vi "copy_from_wrapper.vi"() -> ()   [LabVIEW 2019]
panel:
  in  "Interrupt Run":bool
  out "CMD Error":string
  out "CMD Output":string
  in  "CMD Output":bool
  in  "Help Button":bool
  out "Output Files Path":path caption="selected path"
  in  "Open Button":bool
  out "# Lines Plot":i32
  out "Output File Loaded?":bool
  out "Spec File Loaded":bool
  in  "Save Specs":bool
  out "Vali File Loaded":bool
  in  "Load Spec File":bool
  in  "Load Vali File":bool
  in  "LUA Specification File":path
  in  "LUA Validation File":path
  in  "Validate":bool
  in  "Clear Plot Selection":bool
  in  "Plot":bool
  out "# Lines":i32
  in  "Parameters to Plot":string(tree)="_3"
  in  "Refresh Button":bool
  in  "Parameters":string(tree)="_3"
  in  "Run":bool
  in  "Stop":bool
  # "Biogas Control Panel"
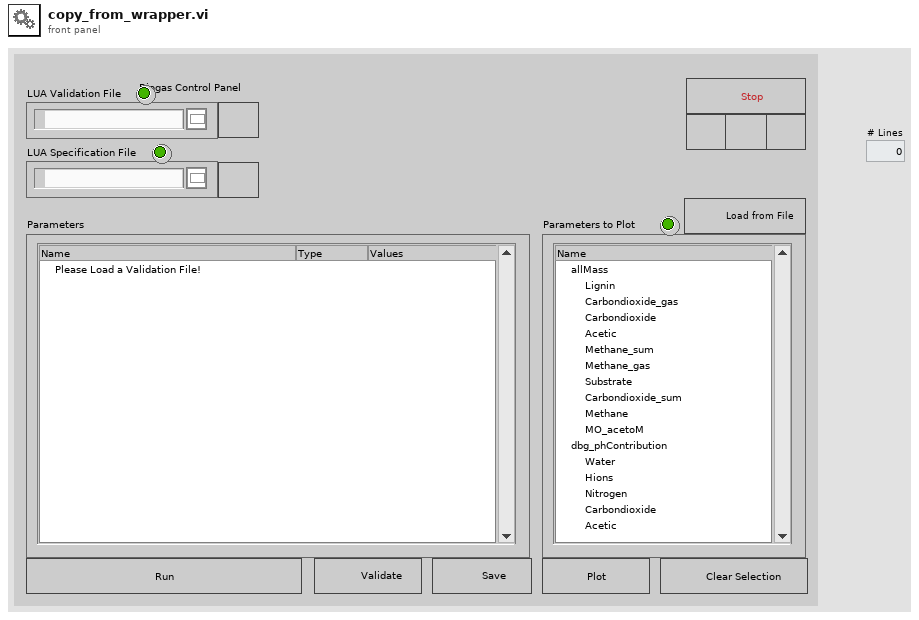
[diagram p1: front panel]
types:
  T1 = typedef "LVPoint32TypeDef.ctl" = cluster{"Horizontal":i32, "Vertical":i32}
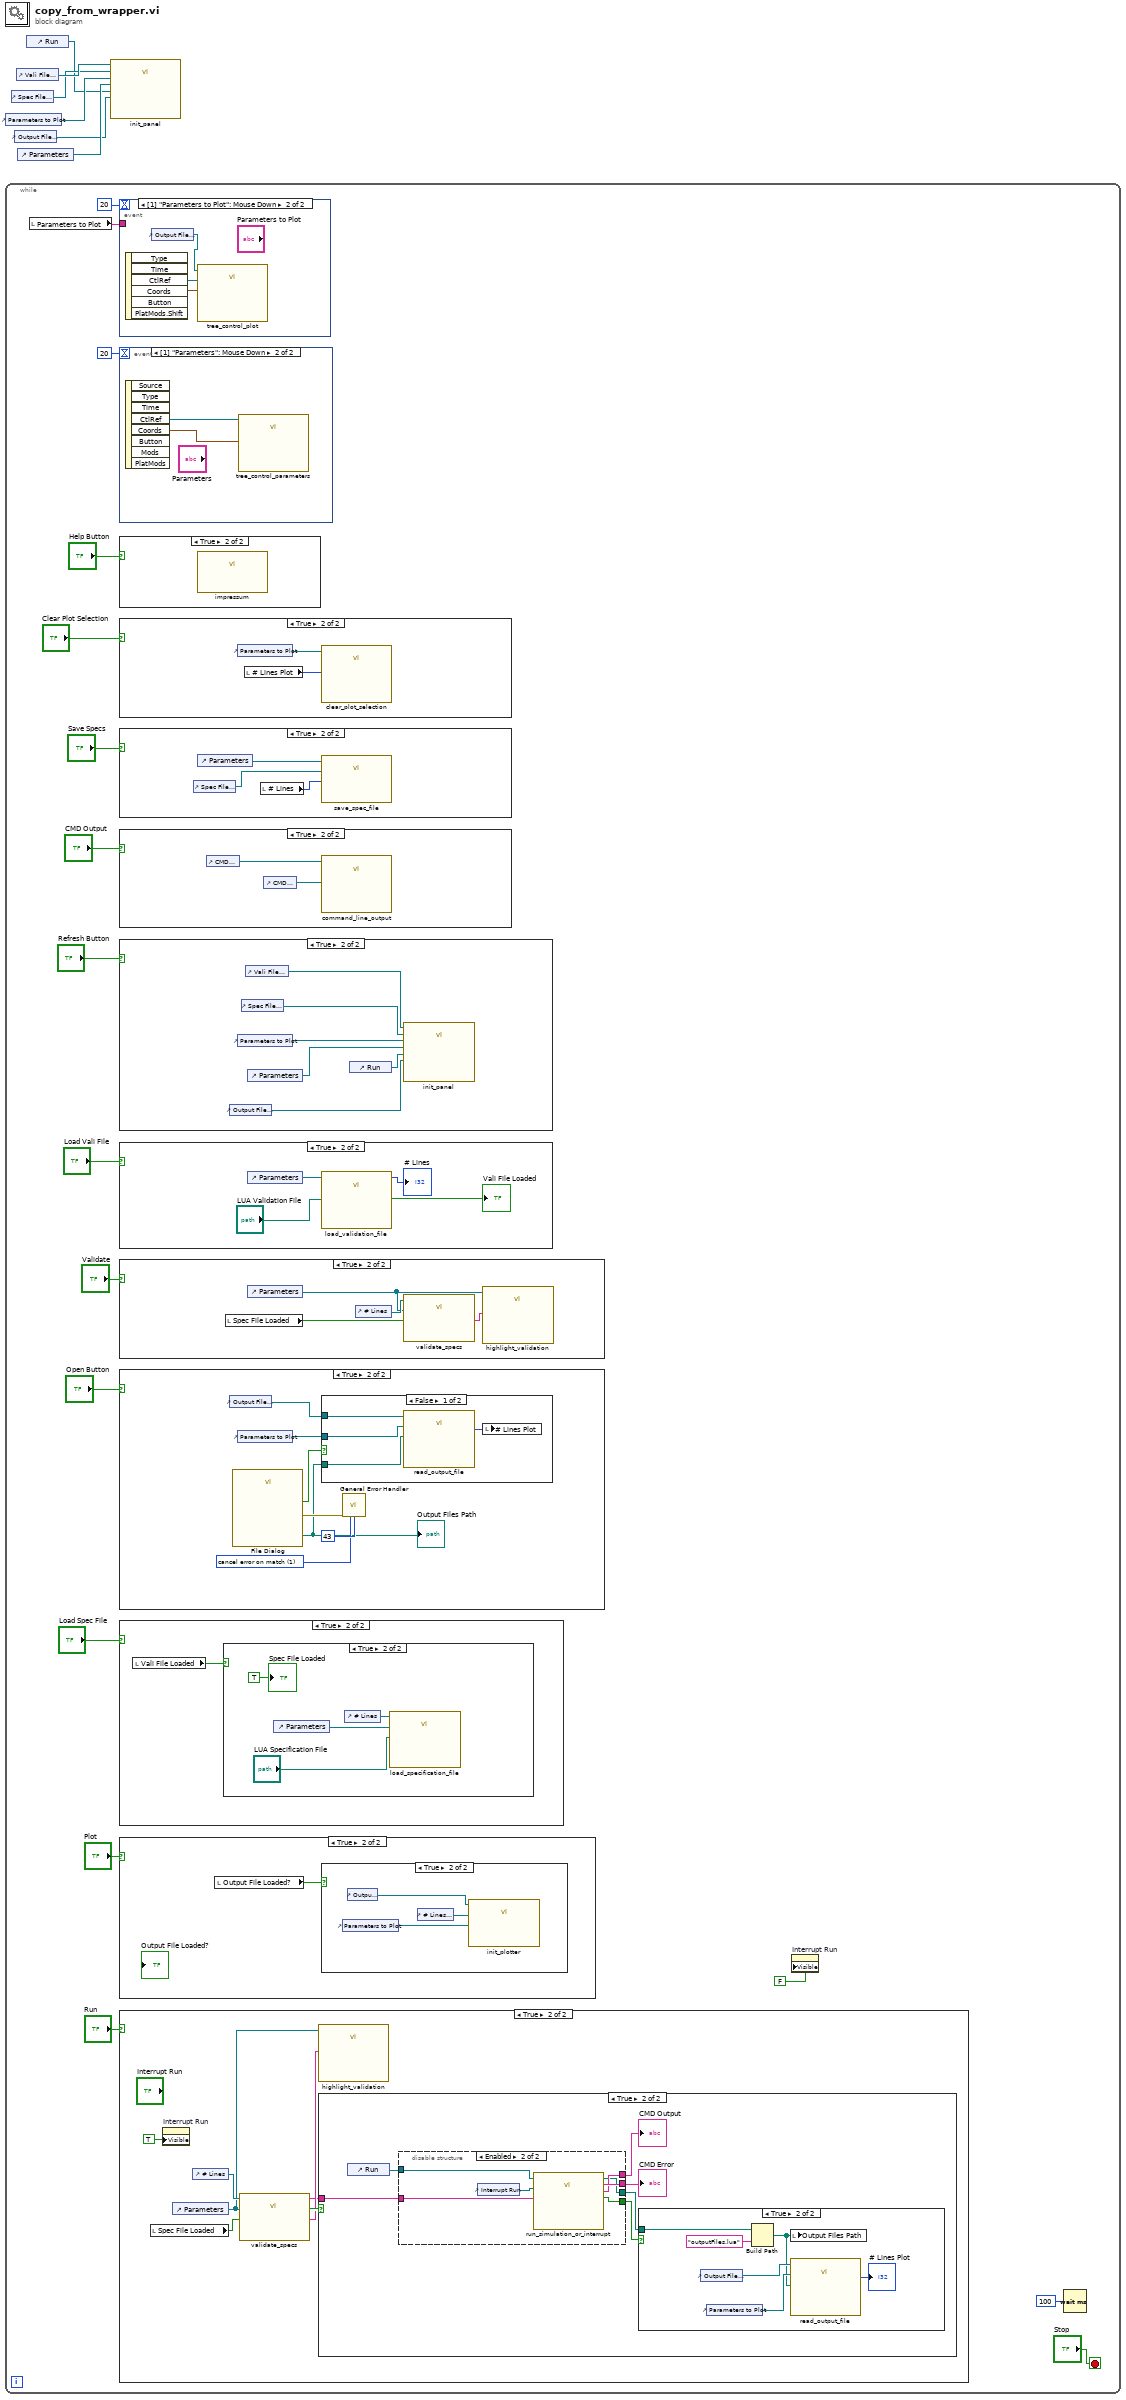
[diagram p0: block diagram]
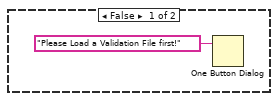
[diagram p9: hidden frame]
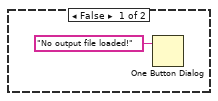
[diagram p12: hidden frame]
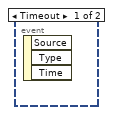
[diagram p13: hidden frame]
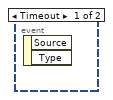
[diagram p15: hidden frame]
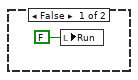
[diagram p18: hidden frame]
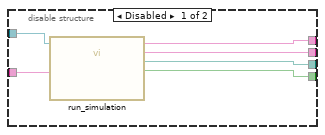
[diagram p19: hidden frame]
diagram:
  n1 = control-ref of="Parameters to Plot"() -> (w4:refnum<vi>)
  n2 = while {
    stop <- "Stop" stop-if-true
    n3 = local read "Parameters to Plot"() -> (w19:string)
    n4 = event shown="[1] \"Parameters to Plot\": Mouse Down" {
      selector: _ -> [_ _]
      dyn-events: _ -> [_ _]
      timeout: 20 -> [_ _]
      tunnel: w19 -> [_ _]
      event Timeout {
        n5 = event-data() -> ()  [unwired: 1 in, 2 out]
      }
      event "Parameters to Plot": Mouse Down {
        n6 = event-data() -> ("CtlRef"=w65:refnum<vi>, "Coords"=w64:T1)  [unwired: 1 in, 4 out]
        n7 = control-ref of="Output File Loaded?"() -> (w63:refnum<vi>)
        n8 = call "tree_control_plot.vi"("Point"=w64, "Plot Tree"=w65, "Output File Loaded?"=w63) -> ()  [unwired: 9 in]
      }
    }
    n9 = event shown="[1] \"Parameters\": Mouse Down" {
      selector: _ -> [_ _]
      dyn-events: _ -> [_ _]
      timeout: 20 -> [_ _]
      event Timeout {
        n10 = event-data() -> ()  [unwired: 1 in, 3 out]
      }
      event "Parameters": Mouse Down {
        n11 = event-data() -> ("CtlRef"=w60:refnum<vi>, "Coords"=w59:T1)  [unwired: 1 in, 6 out]
        n12 = call "tree_control_parameters.vi"("Point"=w59, "Parameters Tree"=w60) -> ()  [unwired: 10 in]
      }
    }
    n13 = case shown="True" "Help Button" {
      frame False {
      }
      frame True {
        n14 = call "impressum.vi"() -> ()  [unwired: 12 in]
      }
    }
    n15 = case shown="True" "Clear Plot Selection" {
      frame False {
      }
      frame True {
        n16 = control-ref of="Parameters to Plot"() -> (w61:refnum<vi>)
        n17 = local read "# Lines Plot"() -> (w62:i32)
        n18 = call "clear_plot_selection.vi"("# Lines Plot"=w62, "Plot Tree"=w61) -> ()  [unwired: 10 in]
      }
    }
    n19 = case shown="True" "Save Specs" {
      frame False {
      }
      frame True {
        n20 = control-ref of="Spec File Loaded"() -> (w37:refnum<vi>)
        n21 = control-ref of="Parameters"() -> (w38:refnum<vi>)
        n22 = local read "# Lines"() -> (w39:i32)
        n23 = call "save_spec_file.vi"("# Lines"=w39, "Spec File Loaded?"=w37, "Parameters Tree"=w38) -> ()  [unwired: 9 in]
      }
    }
    n24 = case shown="True" "CMD Output" {
      frame False {
      }
      frame True {
        n25 = control-ref of="CMD Output"() -> (w24:refnum<vi>)
        n26 = control-ref of="CMD Error"() -> (w25:refnum<vi>)
        n27 = call "command_line_output.vi"("CMD Error"=w25, "CMD Output"=w24) -> ()  [unwired: 10 in]
      }
    }
    n28 = case shown="True" "Refresh Button" {
      frame False {
      }
      frame True {
        n29 = control-ref of="Output File Loaded?"() -> (w67:refnum<vi>)
        n30 = control-ref of="Parameters to Plot"() -> (w69:refnum<vi>)
        n31 = control-ref of="Spec File Loaded"() -> (w68:refnum<vi>)
        n32 = control-ref of="Vali File Loaded"() -> (w71:refnum<vi>)
        n33 = control-ref of="Parameters"() -> (w70:refnum<vi>)
        n34 = control-ref of="Run"() -> (w66:refnum<vi>)
        n35 = call "init_panel.vi"("Run"=w66, "Succesfull Run"=w67, "Parameters Tree"=w70, "Plot Tree"=w69, "Spec File Loaded?"=w68, "Vali File Loaded?"=w71) -> ()  [unwired: 6 in]
      }
    }
    n36 = case shown="True" "Load Vali File" {
      frame False {
      }
      frame True {
        n37 = control-ref of="Parameters"() -> (w52:refnum<vi>)
        n38 = call "load_validation_file.vi"("LUA Validation File"="LUA Validation File", "Parameters Tree"=w52) -> ("Vali File Loaded"=→"Vali File Loaded":bool, "# Lines"=→"# Lines":i32)  [unwired: 8 in]
      }
    }
    n39 = case shown="True" "Validate" {
      frame False {
      }
      frame True {
        n40 = local read "Spec File Loaded"() -> (w43:bool)
        n41 = control-ref of="Parameters"() -> (w40:refnum<vi>)
        n42 = control-ref of="# Lines"() -> (w42:refnum<vi>)
        n43 = call "validate_specs.vi"("Spec File Loaded"=w43, "Parameters Tree"=w40, "# Lines"=w42) -> ("validationErrors"=w41:string)  [unwired: 6 in, 2 out]
        n44 = call "highlight_validation.vi"("validationErrors"=w41, "Parameters Tree"=w40) -> ()  [unwired: 10 in]
      }
    }
    n45 = case shown="True" "Open Button" {
      frame False {
      }
      frame True {
        w30 = 1 items=["no exception", "cancel error on match", "set error on match"] ("[exception action] (none:0)")
        n46 = control-ref of="Output File Loaded?"() -> (w26:refnum<vi>)
        n47 = call "File Dialog"() -> ("selected path"=w28:path, "cancelled"=w29:bool, "error out"=w32:errorcluster)  [unwired: 12 in, 1 out]
        "Output Files Path" <- w28
        n48 = control-ref of="Parameters to Plot"() -> (w27:refnum<vi>)
        n49 = case shown="False" w29 {
          tunnel: w28 -> [w36 _]
          tunnel: w27 -> [w35 _]
          tunnel: w26 -> [w33 _]
          frame False {
            n50 = call "read_output_file.vi"("TMP Filepath"=w36, "Plot Tree"=w35, "Output File Loaded?"=w33) -> ("# Lines Plot"=w34:i32)  [unwired: 8 in]
            n51 = local write "# Lines Plot"(w34) -> ()
          }
          frame True {
          }
        }
        n52 = call <vilib>:"General Error Handler.vi"("error in (no error)"=w32, "[exception action] (none:0)"=w30, "[exception code]"=43) -> ()  [unwired: 8 in, 5 out]
      }
    }
    n53 = case shown="True" "Load Spec File" {
      frame False {
      }
      frame True {
        n54 = local read "Vali File Loaded"() -> (w44:bool)
        n55 = case shown="True" w44 {
          frame False {
            n56 = One Button Dialog(message="Please Load a Validation File first!") -> ()  [unwired: 1 in, 1 out]
          }
          frame True {
            n57 = control-ref of="Parameters"() -> (w47:refnum<vi>)
            n58 = control-ref of="# Lines"() -> (w48:refnum<vi>)
            n59 = call "load_specification_file.vi"("LUA Specification File"="LUA Specification File", "Parameters Tree"=w47, "Digital in"=w48) -> ()  [unwired: 9 in]
            "Spec File Loaded" <- TRUE ("Spec File Loaded")
          }
        }
      }
    }
    n60 = case shown="True" "Plot" {
      frame False {
      }
      frame True {
        n61 = local read "Output File Loaded?"() -> (w54:bool)
        n62 = case shown="True" w54 {
          frame False {
            n63 = One Button Dialog(message="No output file loaded!") -> ()  [unwired: 1 in, 1 out]
          }
          frame True {
            n64 = control-ref of="Parameters to Plot"() -> (w56:refnum<vi>)
            n65 = control-ref of="Output Files Path"() -> (w58:refnum<vi>)
            n66 = control-ref of="# Lines Plot"() -> (w57:refnum<vi>)
            n67 = call "init_plotter.vi"("Plot Tree"=w56, "#Lines Plot"=w57, "Output Files Path"=w58) -> ()  [unwired: 9 in]
          }
        }
      }
    }
    n68 = case shown="True" "Run" {
      frame False {
      }
      frame True {
        n69 = local read "Spec File Loaded"() -> (w77:bool)
        n70 = property on="Interrupt Run" class="Bool (strict)"("Visible"=TRUE) -> ()  [unwired: 2 in, 2 out]
        n71 = control-ref of="Parameters"() -> (w75:refnum<vi>)
        n72 = control-ref of="# Lines"() -> (w78:refnum<vi>)
        n73 = call "validate_specs.vi"("Spec File Loaded"=w77, "Parameters Tree"=w75, "# Lines"=w78) -> ("validationErrors"=w74:string, "Valid?"=w76:bool, "Specifications"=w73:string)  [unwired: 6 in]
        n74 = call "highlight_validation.vi"("validationErrors"=w74, "Parameters Tree"=w75) -> ()  [unwired: 10 in]
        n75 = case shown="True" w76 {
          tunnel: w73 -> [_ w80]
          frame False {
            n76 = local write "Run"(FALSE ("Run")) -> ()
          }
          frame True {
            n77 = control-ref of="Run"() -> (w85:refnum<vi>)
            n78 = disable-structure shown="Enabled" {
              disable-tunnel: w85 -> [w91 w93]
              disable-tunnel: [w90 w95] -> w84
              disable-tunnel: [w89 w96] -> w83
              disable-tunnel: [w88 w97] -> w82
              disable-tunnel: [w87 w98] -> w81
              disable-tunnel: w80 -> [w86 w94]
              frame Disabled {
                n79 = call "run_simulation.vi"("inputSpecs"=w86, "Run"=w91) -> ("OK"=w90:bool, "TMP Filepath"=w89:path, "standard error"=w87:string, "standard output"=w88:string)  [unwired: 6 in]
              }
              frame Enabled {
                n80 = control-ref of="Interrupt Run"() -> (w92:refnum<vi>)
                n81 = call "run_simulation_or_interrupt.vi"("Specifications"=w94, "Interrupt Run"=w92, "Run"=w93) -> ("OK?"=w95:bool, "standard output"=w97:string, "standard error"=w98:string, "TMP Filepath"=w96:path)  [unwired: 5 in]
              }
            }
            "CMD Output" <- w82
            "CMD Error" <- w81
            n82 = case shown="True" w84 {
              tunnel: w83 -> [_ w103]
              frame False {
              }
              frame True {
                n83 = control-ref of="Output File Loaded?"() -> (w100:refnum<vi>)
                n84 = control-ref of="Parameters to Plot"() -> (w104:refnum<vi>)
                n85 = Build Path(base path=w103, name or relative path="outputFiles.lua") -> (appended path=w99:path)
                n86 = local write "Output Files Path"(w99) -> ()
                n87 = call "read_output_file.vi"("TMP Filepath"=w99, "Plot Tree"=w104, "Output File Loaded?"=w100) -> ("# Lines Plot"=→"# Lines Plot":i32)  [unwired: 8 in]
              }
            }
          }
        }
      }
    }
    n88 = property on="Interrupt Run" class="Bool (strict)"("Visible"=FALSE) -> ()  [unwired: 2 in, 2 out]
    n89 = Wait (ms)(milliseconds to wait=u32 100) -> ()  [unwired: 1 out]
  }
  n90 = control-ref of="Spec File Loaded"() -> (w3:refnum<vi>)
  n91 = control-ref of="Output File Loaded?"() -> (w2:refnum<vi>)
  n92 = control-ref of="Vali File Loaded"() -> (w6:refnum<vi>)
  n93 = control-ref of="Parameters"() -> (w5:refnum<vi>)
  n94 = control-ref of="Run"() -> (w1:refnum<vi>)
  n95 = call "init_panel.vi"("Run"=w1, "Succesfull Run"=w2, "Parameters Tree"=w5, "Plot Tree"=w4, "Spec File Loaded?"=w3, "Vali File Loaded?"=w6) -> ()  [unwired: 6 in]
